vi "tcpMessageServer.vi"(9 "Disable Nagle":bool, 11 "server configuration":T1={"client ID"="tcpServer", "remote host"="", "local port"=50001, "remote port"=0}) -> (0 "error out":errorcluster)   [LabVIEW 2014]
doc: "A couple tcpMessageServer and tcpMessageClient ensures communication between two instances. Each one can both transmit or receive CR/LF terminated message strings; however one of the member has to be a Server and the other a Client. Both sit and wait for the other party to connect.\n\nThe difference is: \n* the Server accpts connections on the specified port from any incoming host (the inputs \"remote host\" and \"remote port\" are ignored) \n* the Client must know to which host is directed\n\nCommunication with them, while running, is done via four named queues. One acts as a transmission buffer, another as a receive buffer; one is a single element queue, which cause the shutdown of the actor when a True is enqueued to it; the last one is a read only one-element queue which reports the actor status."
uses:
  typedefs/clientStatus.ctl
  typedefs/clientConfiguration.ctl
panel:
  in  "manual shutdown":bool
  out "remote address":string
  out "remote port":u16
  out "string to send":string
  out "received string":string
  out "status":T2
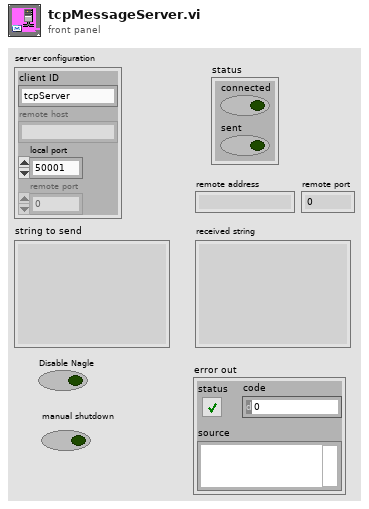
[diagram p1: front panel]
types:
  T1 = typedef "clientConfiguration.ctl" = cluster{"client ID":string, "remote host":string, "local port":u16, "remote port":u16}
  T2 = typedef "clientStatus.ctl" = cluster{"connected":bool, "sent":bool}
  T3 = typedef "QueueCluster.ctl" = cluster{"status":cluster{"queue":refnum<queue>, "error out":errorcluster}, "receive":cluster{"queue":refnum<queue>, "error out":errorcluster}, "transmit":cluster{"queue":refnum<queue>, "error out":errorcluster}, "shutdown":cluster{"queue":refnum<queue>, "error out":errorcluster}, "semaphore":T4}
  T4 = typedef "Semaphore RefNum" = refnum<k1>
  T5 = cluster{"queue":refnum<queue>, "error out":errorcluster}
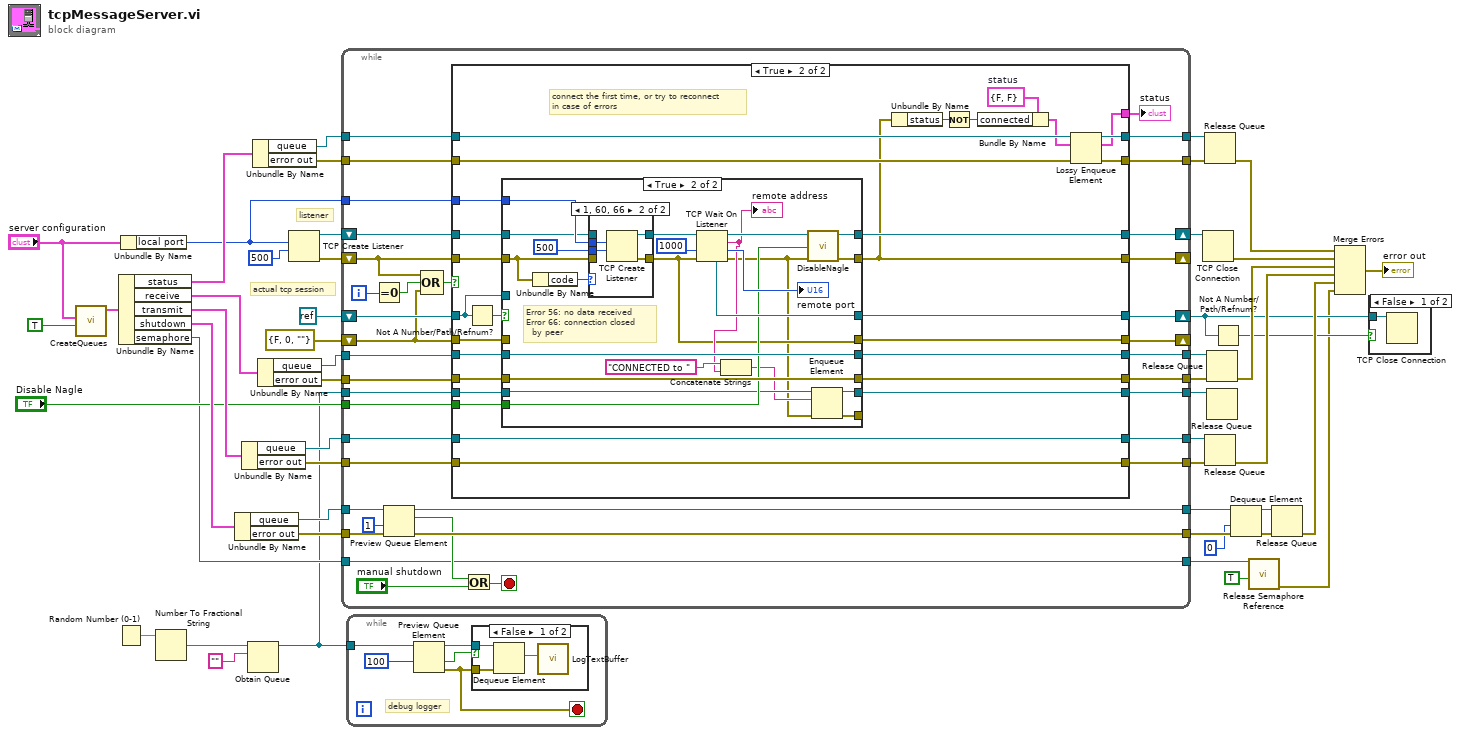
[diagram p0: block diagram]
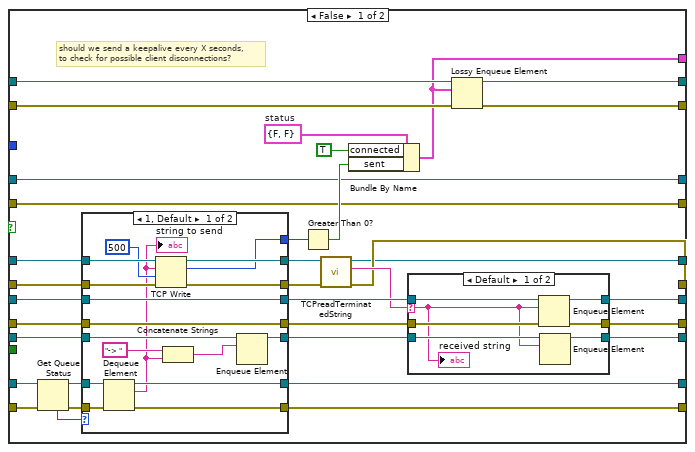
[diagram p4: hidden frame]
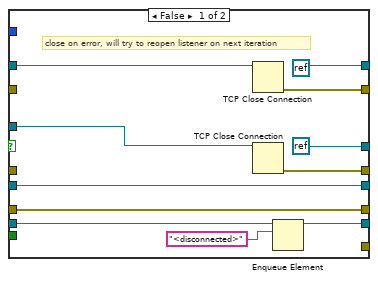
[diagram p7: hidden frame]
diagram:
  # "listener"
  # "actual tcp session"
  n1 = call "CreateQueues.vi"("create if not found? (T)"=TRUE, "client configuration"="server configuration") -> ("output cluster"=w19:T3)  [unwired: 8 in, 1 out]
  n2 = Random Number (0-1)() -> (number: 0 to 1=w4:dbl)
  n3 = Unbundle By Name(w19) -> ("status"=w49:T5, "receive"=w46:T5, "transmit"=w45:T5, "shutdown"=w40:T5, "semaphore"=w9:T4)
  n4 = Unbundle By Name("server configuration") -> ("local port"=w24:u16)
  n5 = Number To Fractional String(number=w4) -> (F-format string=w5:string)  [unwired: 3 in]
  n6 = Unbundle By Name(w40) -> ("queue"=w41:refnum<queue>, "error out"=w42:errorcluster)
  n7 = Unbundle By Name(w45) -> ("queue"=w44:refnum<queue>, "error out"=w43:errorcluster)
  n8 = Obtain Queue(name (unnamed)=w5, element data type="" ("source")) -> (queue out=w2:refnum<queue>)  [unwired: 3 in, 2 out]
  n9 = Unbundle By Name(w49) -> ("queue"=w50:refnum<queue>, "error out"=w51:errorcluster)
  n10 = Unbundle By Name(w46) -> ("queue"=w47:refnum<queue>, "error out"=w48:errorcluster)
  n11 = TCP Create Listener(9:500 ("timeout ms (25000)"), 10:w24) -> (0:w27:errorcluster, 3:w28:refnum<k5>)  [unwired: 3 in, 1 out]
  n12 = while {
    shift-right: [w86] -> _
    shift-left: w27 -> [w85]
    shift-right: [w87] -> w29
    shift-left: w28 -> [w88]
    tunnel: w42 -> [w63]
    tunnel: w41 -> [w64]
    tunnel: w50 -> [w81]
    tunnel: w51 -> [w80]
    tunnel: w47 -> [w79]
    tunnel: w48 -> [w78]
    tunnel: w44 -> [w77]
    tunnel: w43 -> [w76]
    tunnel: [w62] -> w17
    tunnel: [w61] -> w15
    tunnel: [w75] -> w30
    tunnel: [w74] -> w31
    tunnel: [w72] -> w32
    tunnel: [w71] -> w33
    tunnel: [w70] -> w34
    tunnel: [w69] -> w35
    shift-right: [w66] -> w22
    shift-left: refnum<k0> refnum -> [w67]
    tunnel: w24 -> [w68]
    shift-right: [w65] -> _
    shift-left: errorcluster {"status"=FALSE, "code"=0, "source"=""} ("error out") -> [w58]
    tunnel: "Disable Nagle" -> [w55]
    tunnel: w9 -> [w54]
    tunnel: [w54] -> w8
    tunnel: w2 -> [w53]
    tunnel: [w52] -> w1
    i -> [w84]
    stop <- w57 stop-if-true
    n13 = Equal To 0?(x=w84) -> (x = 0?=w83:bool)
    n14 = Preview Queue Element(queue=w64, timeout in ms (-1)=1, error in (no error)=w63) -> (queue out=w62:refnum<queue>, element=w60:bool, error out=w61:errorcluster)  [unwired: 1 out]
    n15 = Compound Arithmetic op=OR(w85, w83, w58) -> (w82:bool)
    n16 = case shown="True" w82 {
      tunnel: w88 -> [w98 w174]
      tunnel: [w98 w171] -> w87
      tunnel: [w97 w164] -> w86
      tunnel: w85 -> [w97 w175]
      tunnel: w81 -> [w122 w183]
      tunnel: w80 -> [w121 w182]
      tunnel: w79 -> [w108 w170]
      tunnel: w78 -> [w107 w169]
      tunnel: w77 -> [w116 w179]
      tunnel: w76 -> [w115 w178]
      tunnel: [w120 w181] -> w75
      tunnel: [w119 w180] -> w74
      tunnel: [w111 w162] -> w73
      tunnel: [w102 w168] -> w72
      tunnel: [w101 w167] -> w71
      tunnel: [w110 w179] -> w70
      tunnel: [w109 w178] -> w69
      tunnel: w68 -> [_ w176]
      tunnel: w67 -> [w100 w173]
      tunnel: [w92 w172] -> w66
      tunnel: w58 -> [w99 w166]
      tunnel: [w93 w165] -> w65
      tunnel: w55 -> [_ w159]
      tunnel: w53 -> [w91 w158]
      tunnel: [w90 w157] -> w52
      frame False {
        w118 = T2 {"connected"=FALSE, "sent"=FALSE}  # status
        # "should we send a keepalive every X seconds,\nto check for possible client disconnections?"
        n17 = Get Queue Status(queue=w116, error in (no error)=w115) -> (queue out=w113:refnum<queue>, error out=w112:errorcluster, # elements in queue=w114:i32)  [unwired: 1 in, 5 out]
        n18 = case shown="1, Default" w114 {
          tunnel: w113 -> [w149 w152]
          tunnel: w112 -> [w148 w151]
          tunnel: [w147 w152] -> w110
          tunnel: [w146 w151] -> w109
          tunnel: w108 -> [w145 w156]
          tunnel: w107 -> [w144 w155]
          tunnel: [w145 w156] -> w104
          tunnel: [w144 w155] -> w103
          tunnel: w100 -> [w143 w154]
          tunnel: w99 -> [w142 w153]
          tunnel: [w141 w154] -> w95
          tunnel: [w140 w153] -> w96
          tunnel: [w139 _] -> w106
          tunnel: w91 -> [w136 w150]
          tunnel: [w137 w150] -> w89
          frame 1, Default {
            n19 = Dequeue Element(queue=w149, error in (no error)=w148) -> (queue out=w147:refnum<queue>, element=w133:string, error out=w146:errorcluster)  [unwired: 1 in, 1 out]
            "string to send" <- w133
            n20 = TCP Write(connection ID=w143, data in=w133, error in (no error)=w142, 9:500 ("timeout ms (25000)")) -> (connection ID out=w141:refnum<k5>, bytes written=w139:i32, error out=w140:errorcluster)
            n21 = Concatenate Strings("-> " ("string"), w133) -> (w134:string)
            n22 = Enqueue Element(queue=w136, element=w134) -> (queue out=w137:refnum<queue>)  [unwired: 2 in, 2 out]
          }
          frame 0 {
          }
        }
        n23 = Greater Than 0?(x=w106) -> (x > 0?=w105:bool)
        n24 = call "TCPreadTerminatedString.vi"("error in (no error)"=w96, "TCP Network Connection in"=w95) -> ("error out"=w93:errorcluster, "string out"=w94:string, "TCP Network Connection out"=w92:refnum<k5>)  [unwired: 7 in]
        n25 = Bundle By Name(cluster=w118, "connected"=TRUE, "sent"=w105) -> (w111:T2)
        n26 = case shown="Default" w94 {
          selector: w94 -> [w123 _]
          tunnel: w104 -> [w127 w132]
          tunnel: w103 -> [w126 w131]
          tunnel: [w129 w132] -> w102
          tunnel: [w128 w131] -> w101
          tunnel: [w125 w130] -> w90
          tunnel: w89 -> [w124 w130]
          frame Default {
            n27 = Enqueue Element(queue=w127, element=w123, error in (no error)=w126) -> (queue out=w129:refnum<queue>, error out=w128:errorcluster)  [unwired: 1 in, 1 out]
            n28 = Enqueue Element(queue=w124, element=w123) -> (queue out=w125:refnum<queue>)  [unwired: 2 in, 2 out]
            "received string" <- w123
          }
          frame "" {
          }
        }
        n29 = Lossy Enqueue Element(queue=w122, element=w111, error in (no error)=w121) -> (queue out=w120:refnum<queue>, error out=w119:errorcluster)  [unwired: 2 out]
      }
      frame True {
        w163 = T2 {"connected"=FALSE, "sent"=FALSE}  # status
        # "connect the first time, or try to reconnect\nin case of errors"
        n30 = Not A Number/Path/Refnum?(number/path/refnum=w173) -> (NaN/Path/Refnum?=w177:bool)
        n31 = case shown="True" w177 {
          tunnel: w174 -> [w192 w211]
          tunnel: w175 -> [_ w210]
          tunnel: [refnum<k0> refnum w206] -> w171
          tunnel: [w188 w205] -> w164
          tunnel: [refnum<k0> refnum w215] -> w172
          tunnel: w173 -> [w194 _]
          tunnel: w176 -> [_ w213]
          tunnel: w170 -> [w190 w209]
          tunnel: w169 -> [w189 w208]
          tunnel: [w190 w209] -> w168
          tunnel: [w189 w208] -> w167
          tunnel: w166 -> [_ _]
          tunnel: [w187 w197] -> w165
          tunnel: w159 -> [_ w203]
          tunnel: w158 -> [w185 w201]
          tunnel: [w186 w202] -> w157
          tunnel: [_ w195] -> _
          frame False {
            # "close on error, will try to reopen listener on next iteration"
            n32 = TCP Close Connection(connection ID=w192) -> (error out=w188:errorcluster)  [unwired: 2 in, 1 out]
            n33 = TCP Close Connection(connection ID=w194) -> (error out=w187:errorcluster)  [unwired: 2 in, 1 out]
            n34 = Enqueue Element(queue=w185, element="<disconnected>") -> (queue out=w186:refnum<queue>)  [unwired: 2 in, 2 out]
          }
          frame True {
            # "Error 56: no data received\nError 66: connection closed\n  by peer"
            n35 = Unbundle By Name(w210) -> ("code"=w214:i32)
            n36 = case shown="1, 60, 66" w214 {
              tunnel: w213 -> [_ w222]
              tunnel: [w218 w221] -> w212
              tunnel: w211 -> [w218 _]
              tunnel: [_ w220] -> w197
              tunnel: w210 -> [_ _]
              tunnel: 500 -> [_ w219]
              frame 0, Default {
              }
              frame 1, 60, 66 {
                n37 = TCP Create Listener(9:w219, 10:w222) -> (0:w220:errorcluster, 3:w221:refnum<k5>)  [unwired: 3 in, 1 out]
              }
            }
            n38 = TCP Wait On Listener(8:w197, 9:1000, 11:w212) -> (0:w196:errorcluster, 1:→"remote port":u16, 2:w198:string, 3:w204:refnum<k5>, 4:w215:refnum<k5>)  [unwired: 1 in]
            "remote address" <- w198
            n39 = Concatenate Strings("CONNECTED to " ("new message"), w198) -> (w199:string)
            n40 = call "DisableNagle.vi"("error in"=w196, "TCP_NODELAY"=w203, "connection ID"=w204) -> ("error out"=w205:errorcluster, "connID out"=w206:refnum<k5>)  [unwired: 7 in]
            n41 = Enqueue Element(queue=w201, element=w199, error in (no error)=w196) -> (queue out=w202:refnum<queue>, error out=w195:errorcluster)  [unwired: 1 in, 1 out]
          }
        }
        n42 = Unbundle By Name(w164) -> ("status"=w161:bool)
        n43 = Not(x=w161) -> (.not. x?=w160:bool)
        n44 = Bundle By Name(cluster=w163, "connected"=w160) -> (w162:T2)
        n45 = Lossy Enqueue Element(queue=w183, element=w162, error in (no error)=w182) -> (queue out=w181:refnum<queue>, error out=w180:errorcluster)  [unwired: 2 out]
      }
    }
    "status" <- w73
    n46 = Or(x=w60, y="manual shutdown") -> (x .or. y?=w57:bool)
  }
  n47 = while {
    tunnel: w2 -> [w226]
    stop <- w223 stop-if-true
    # "debug logger"
    n48 = Preview Queue Element(queue=w226, timeout in ms (-1)=100) -> (queue out=w227:refnum<queue>, timed out?=w224:bool, error out=w223:errorcluster)  [unwired: 1 in, 1 out]
    n49 = case shown="False" w224 {
      tunnel: w227 -> [w229 _]
      tunnel: w223 -> [w228 _]
      frame False {
        n50 = Dequeue Element(queue=w229, error in (no error)=w228) -> (element=w230:string)  [unwired: 1 in, 3 out]
        n51 = call "LogTextBuffer.vi"("new message"=w230) -> ()  [unwired: 10 in, 1 out]
      }
      frame True {
      }
    }
  }
  n52 = TCP Close Connection(connection ID=w29) -> (error out=w12:errorcluster)  [unwired: 2 in, 1 out]
  n53 = Release Queue(queue=w30, error in (no error)=w31) -> (error out=w13:errorcluster)  [unwired: 1 in, 2 out]
  n54 = Release Queue(queue=w34, error in (no error)=w35) -> (error out=w37:errorcluster)  [unwired: 1 in, 2 out]
  n55 = Release Queue(queue=w32, error in (no error)=w33) -> (error out=w36:errorcluster)  [unwired: 1 in, 2 out]
  n56 = Release Queue(queue=w1) -> ()  [unwired: 2 in, 3 out]
  n57 = Not A Number/Path/Refnum?(number/path/refnum=w22) -> (NaN/Path/Refnum?=w23:bool)
  n58 = Dequeue Element(queue=w17, timeout in ms (-1)=0, error in (no error)=w15) -> (queue out=w16:refnum<queue>, error out=w14:errorcluster)  [unwired: 2 out]
  n59 = call <vilib>:"Release Semaphore Reference.vi"("force destroy? (F)"=TRUE, "semaphore"=w8) -> ("error out"=w7:errorcluster)  [unwired: 8 in, 1 out]
  n60 = Release Queue(queue=w16, error in (no error)=w14) -> (error out=w38:errorcluster)  [unwired: 1 in, 2 out]
  n61 = Merge Errors(w13, w12, w36, w37, w38, w7) -> (→"error out":errorcluster)
  n62 = case shown="False" w23 {
    tunnel: w22 -> [w231 _]
    frame False {
      n63 = TCP Close Connection(connection ID=w231) -> ()  [unwired: 2 in, 2 out]
    }
    frame True {
    }
  }
